vi "Recursive File List2.vi"(4 "Folders to Exclude\nREP ( ^[_.] as Default)\nempty to disable this feature":string="^[_.]", 6 "pattern":string, 8 "error in (no error)":errorcluster, 9 "Continue Recursing on Error? (F)":bool, 10 "Treat LLBs as Folders?":bool, 11 "Folder Path":path) -> (0 "error out":errorcluster, 1 "Number of Files":i32, 2 "All Files in Dir":path[](array[path]), 3 "dup Folder Path":path, 5 "All Folders":path[](array[path]))   [LabVIEW 2017]
doc: "Lists the contents of a folder or LLB."
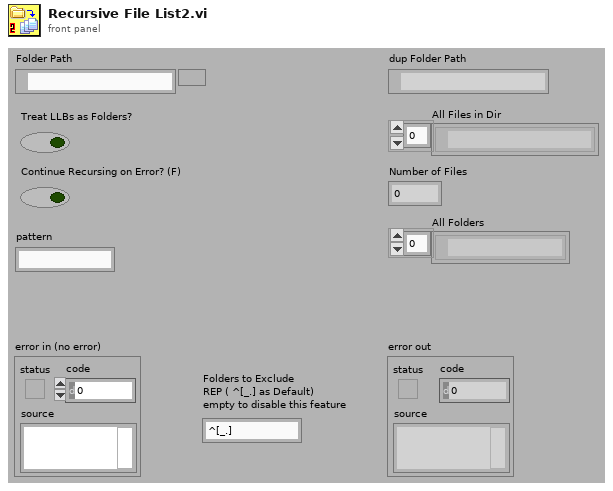
[diagram p1: front panel]
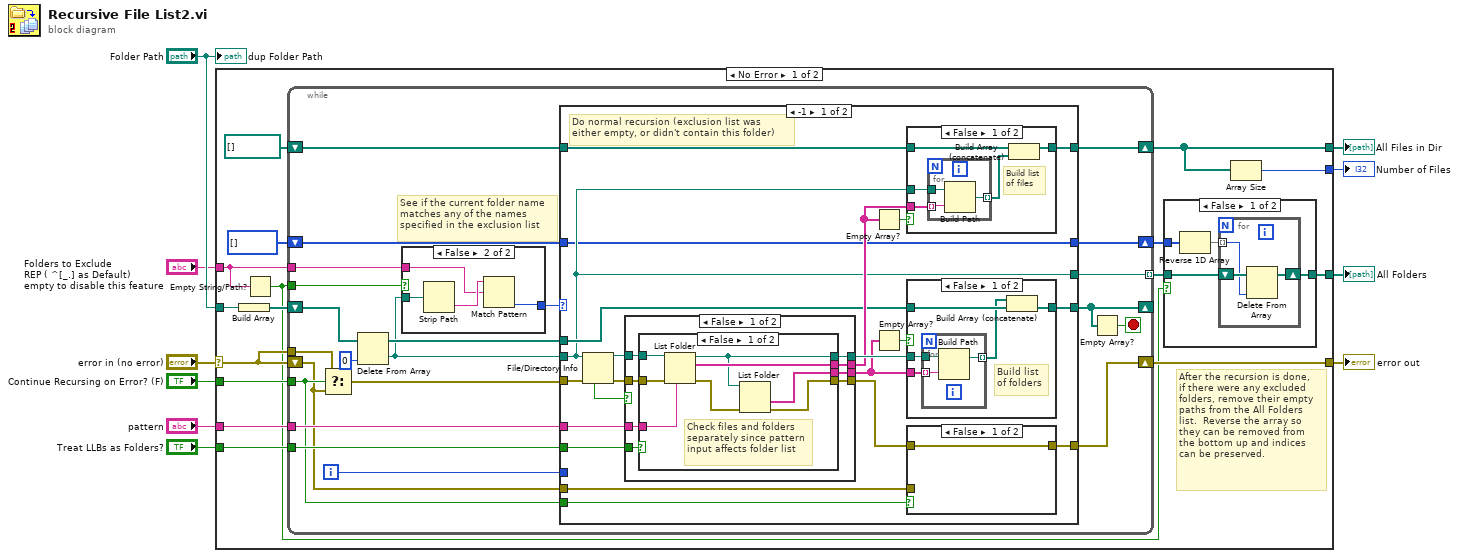
[diagram p0: block diagram]
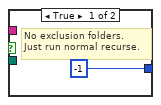
[diagram p3: hidden frame]
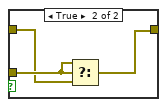
[diagram p5: hidden frame]
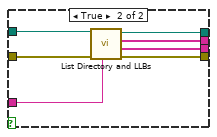
[diagram p6: hidden frame]
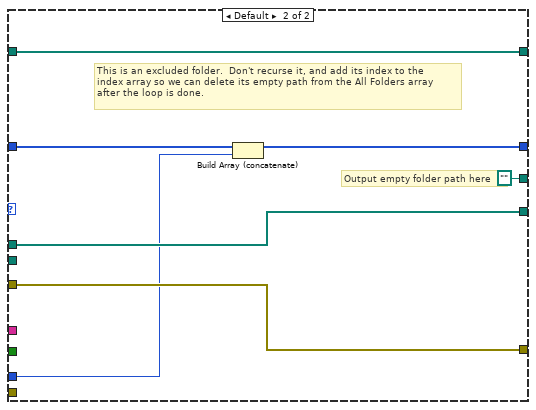
[diagram p9: hidden frame]
diagram:
  n1 = case shown="No Error" "error in (no error)" {
    selector: "error in (no error)" -> [w17 w137]
    tunnel: "Folder Path" -> [w26 _]
    tunnel: [w20 _] -> w10
    tunnel: [w19 _] -> w9
    tunnel: [w21 w137] -> w8
    tunnel: "Treat LLBs as Folders?" -> [w23 _]
    tunnel: [w12 _] -> w5
    tunnel: "pattern" -> [w22 _]
    tunnel: "Continue Recursing on Error? (F)" -> [w18 _]
    tunnel: "Folders to Exclude\nREP ( ^[_.] as Default)\nempty to disable this feature" -> [w15 _]
    frame No Error {
      # "After the recursion is done,\nif there were any excluded\nfolders, remove their empty\npaths from the All Folders\nlist.  Reverse the array so\nthey can be removed from\nthe bottom up and indices\ncan be preserved."
      n2 = Build Array(w26) -> (w25:path[])
      n3 = Empty String/Path?(string/path=w15) -> (empty?=w13:bool)
      n4 = while {
        shift-left: path[] [] ("Array Constant") -> [w54]
        shift-right: [w56] -> w20
        shift-left: w25 -> [w55]
        shift-right: [w51] -> _
        shift-right: [w45] -> w21
        shift-left: w17 -> [w44]
        tunnel: w23 -> [w53]
        tunnel: [w41] -> w14 mode=indexing
        tunnel: w22 -> [w52]
        tunnel: w18 -> [w46]
        tunnel: w17 -> [w47]
        tunnel: w15 -> [w37]
        shift-right: [w40] -> w11
        shift-left: i32[] [] -> [w42]
        tunnel: w13 -> [w38]
        i -> [w39]
        stop <- w50 stop-if-true
        # "See if the current folder name\nmatches any of the names\nspecified in the exclusion list"
        n5 = Select(t=w47, s=w46, f=w44) -> (s? t:f=w48:errorcluster)
        n6 = Delete From Array(array=w55, index=0) -> (deleted portion=w36:path, array with subset deleted=w43:path[])  [unwired: 1 in]
        n7 = case shown="False" w38 {
          tunnel: w37 -> [_ w58]
          tunnel: w36 -> [_ w61]
          tunnel: [-1 ("index of element") w60] -> w35
          frame True {
            # "No exclusion folders.\nJust run normal recurse."
          }
          frame False {
            n8 = Strip Path(path=w61) -> (name=w59:string)  [unwired: 1 out]
            n9 = Match Pattern(string=w59, regular expression=w58) -> (offset past match=w60:i32)  [unwired: 1 in, 3 out]
          }
        }
        n10 = case shown="-1" w35 {
          tunnel: [w82 w136] -> w56
          tunnel: w54 -> [w81 w136]
          tunnel: w53 -> [w79 _]
          tunnel: w52 -> [w78 _]
          tunnel: [w75 w135] -> w51
          tunnel: w36 -> [w63 _]
          tunnel: w48 -> [w71 w134]
          tunnel: w46 -> [w69 _]
          tunnel: [w68 w134] -> w45
          tunnel: w44 -> [w67 _]
          tunnel: w43 -> [w64 w135]
          tunnel: w42 -> [w62 w133]
          tunnel: [w63 path ""] -> w41
          tunnel: [w62 w132] -> w40
          tunnel: w39 -> [_ w131]
          frame -1 {
            # "Do normal recursion (exclusion list was\neither empty, or didn't contain this folder)"
            n11 = File/Directory Info(path=w63, error in=w71) -> (path out=w73:path, error out=w74:errorcluster, shortcut=w72:bool)  [unwired: 4 out]
            n12 = case shown="False" w72 {
              tunnel: [w103 _] -> w65
              tunnel: [w102 w120] -> w80
              tunnel: [w101 w119] -> w70
              tunnel: w79 -> [w100 _]
              tunnel: w78 -> [w99 _]
              tunnel: [w98 _] -> w77
              tunnel: w74 -> [w97 w119]
              tunnel: w73 -> [w96 w120]
              frame False {
                n13 = case shown="False" w100 {
                  tunnel: [w111 w115] -> w103
                  tunnel: [w105 w114] -> w98
                  tunnel: w96 -> [w110 w118]
                  tunnel: [w104 w116] -> w102
                  tunnel: [w106 w113] -> w101
                  tunnel: w97 -> [w109 w117]
                  tunnel: w99 -> [w108 w112]
                  frame False {
                    # "Check files and folders\nseparately since pattern\ninput affects folder list"
                    n14 = List Folder(path=w110, pattern=w108, error in=w109) -> (path out=w104:path, filenames=w111:string[], error out=w107:errorcluster)  [unwired: 2 out]
                    n15 = List Folder(path=w104, error in=w107) -> (folder names=w105:string[], error out=w106:errorcluster)  [unwired: 4 out]
                  }
                  frame True {
                    n16 = call <vilib>:"List Directory and LLBs.vi"("pattern"=w112, "error in (no error)"=w117, "Folder Path"=w118) -> ("error out"=w113:errorcluster, "Folders and LLBs"=w114:string[], "Files sans LLBs"=w115:string[], "dup Folder Path"=w116:path)  [unwired: 5 out]
                  }
                }
              }
              frame True {
                # "Do not attempt to recurse the contents\nof folder shortcuts"
              }
            }
            n17 = Empty Array?(array=w65) -> (empty?=w66:bool)
            n18 = Empty Array?(array=w77) -> (empty?=w76:bool)
            n19 = case shown="False" w66 {
              tunnel: [w87 w91] -> w82
              tunnel: w65 -> [w86 _]
              tunnel: w81 -> [w85 w91]
              tunnel: w63 -> [w83 _]
              frame False {
                # "Build list of files"
                n20 = for {
                  tunnel: w86 -> [w89] mode=indexing
                  tunnel: w83 -> [w90]
                  tunnel: [w88] -> w84 mode=indexing
                  n21 = Build Path(base path=w90, name or relative path=w89) -> (appended path=w88:path)
                }
                n22 = Build Array (concatenate)(w85, w84) -> (w87:path[])
              }
              frame True {
              }
            }
            n23 = case shown="False" w76 {
              tunnel: w64 -> [w123 w129]
              tunnel: [w124 w129] -> w75
              tunnel: w80 -> [w125 _]
              tunnel: w77 -> [w121 _]
              frame False {
                # "Build list\nof folders"
                n24 = for {
                  tunnel: w125 -> [w128]
                  tunnel: [w127] -> w122 mode=indexing
                  tunnel: w121 -> [w126] mode=indexing
                  n25 = Build Path(base path=w128, name or relative path=w126) -> (appended path=w127:path)
                }
                n26 = Build Array (concatenate)(w122, w123) -> (w124:path[])
              }
              frame True {
              }
            }
            n27 = case shown="False" w69 {
              tunnel: w70 -> [w92 w94]
              tunnel: [w92 w93] -> w68
              tunnel: w67 -> [_ w95]
              frame False {
              }
              frame True {
                n28 = Select(t=w95, s=w95, f=w94) -> (s? t:f=w93:errorcluster)
              }
            }
          }
          frame Default {
            # "Output empty folder path here"
            # "This is an excluded folder.  Don't recurse it, and add its index to the\nindex array so we can delete its empty path from the All Folders array\nafter the loop is done."
            n29 = Build Array (concatenate)(w133, w131) -> (w132:i32[])
          }
        }
        n30 = Empty Array?(array=w51) -> (empty?=w50:bool)
      }
      n31 = case shown="False" w13 {
        tunnel: w14 -> [w29 w34]
        tunnel: [w28 w34] -> w12
        tunnel: w11 -> [w30 _]
        frame False {
          n32 = Reverse 1D Array(array=w30) -> (reversed array=w27:i32[])
          n33 = for {
            shift-right: [w32] -> w28
            shift-left: w29 -> [w33]
            tunnel: w27 -> [w31] mode=indexing
            n34 = Delete From Array(array=w33, index=w31) -> (array with subset deleted=w32:path[])  [unwired: 1 in, 1 out]
          }
        }
        frame True {
          # "No excluded folders.\nDon't run the code that\ndeletes excluded folder\nindices."
        }
      }
      n35 = Array Size(array=w20) -> (size(s)=w19:i32)
    }
    frame Error {
    }
  }
  "All Files in Dir" <- w10
  "Number of Files" <- w9
  "error out" <- w8
  "All Folders" <- w5
  "dup Folder Path" <- "Folder Path"
